vi "ReloadPositions.vi"(6 "Load Positions":dbl[](array[numeric]), 8 "error In":errorcluster, 9 "Device Address In":i32, 10 "DeviceKey In":string="192.168.14.151", 11 "CmdLib In":refnum<k24>) -> (0 "error Out":errorcluster, 1 "Device Address Out":i32, 2 "DeviceKey Out":string, 3 "CmdLib Out":refnum<k24>)   [LabVIEW 2020]
uses:
  C:/GEECS/Developers Version/builds/Device builds/Picomotor8742dotNet/CmdLib.dll
  CmdLib.dll
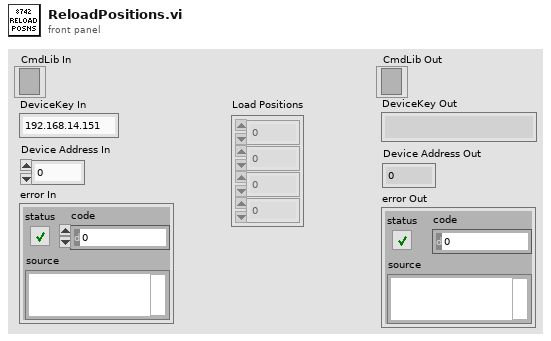
[diagram p1: front panel]
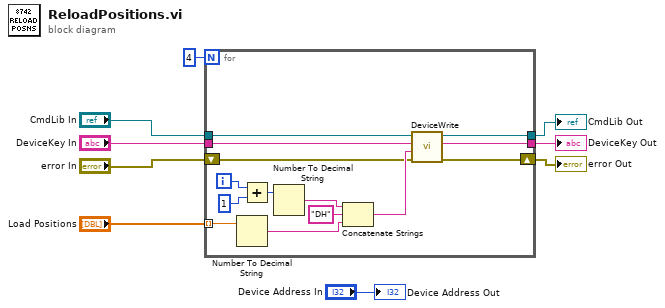
[diagram p0: block diagram]
diagram:
  n1 = for {
    N: 4 -> [_]
    tunnel: "Load Positions" -> [w17] mode=indexing
    tunnel: "DeviceKey In" -> [w13]
    tunnel: "CmdLib In" -> [w12]
    tunnel: [w11] -> w4
    tunnel: [w10] -> w3
    shift-right: [w15] -> w2
    shift-left: "error In" -> [w14]
    i -> [w20]
    n2 = Number To Decimal String(number=w17) -> (decimal integer string=w18:string)  [unwired: 1 in]
    n3 = Add(x=w20, y=1) -> (x+y=w21:i32)
    n4 = Number To Decimal String(number=w21) -> (decimal integer string=w23:string)  [unwired: 1 in]
    n5 = Concatenate Strings(w23, "DH" ("string"), w18) -> (w16:string)
    n6 = call "DeviceWrite.vi"("error in (no error)"=w14, "Command"=w16, "DeviceKey In"=w13, "CmdLib In"=w12) -> ("error out"=w15:errorcluster, "DeviceKey Out"=w10:string, "CmdLib Out"=w11:refnum<k24>)  [unwired: 1 in]
  }
  "CmdLib Out" <- w4
  "DeviceKey Out" <- w3
  "error Out" <- w2
  "Device Address Out" <- "Device Address In"
